vi "Untitled 4.vi"() -> ()   [LabVIEW 2021]
panel:
  out "length":i32
  out "data string":string
  out "result 2":i32
  in  "Array":string[](array[string])
  out "result":i32
  out "appended array":string[](array[string])
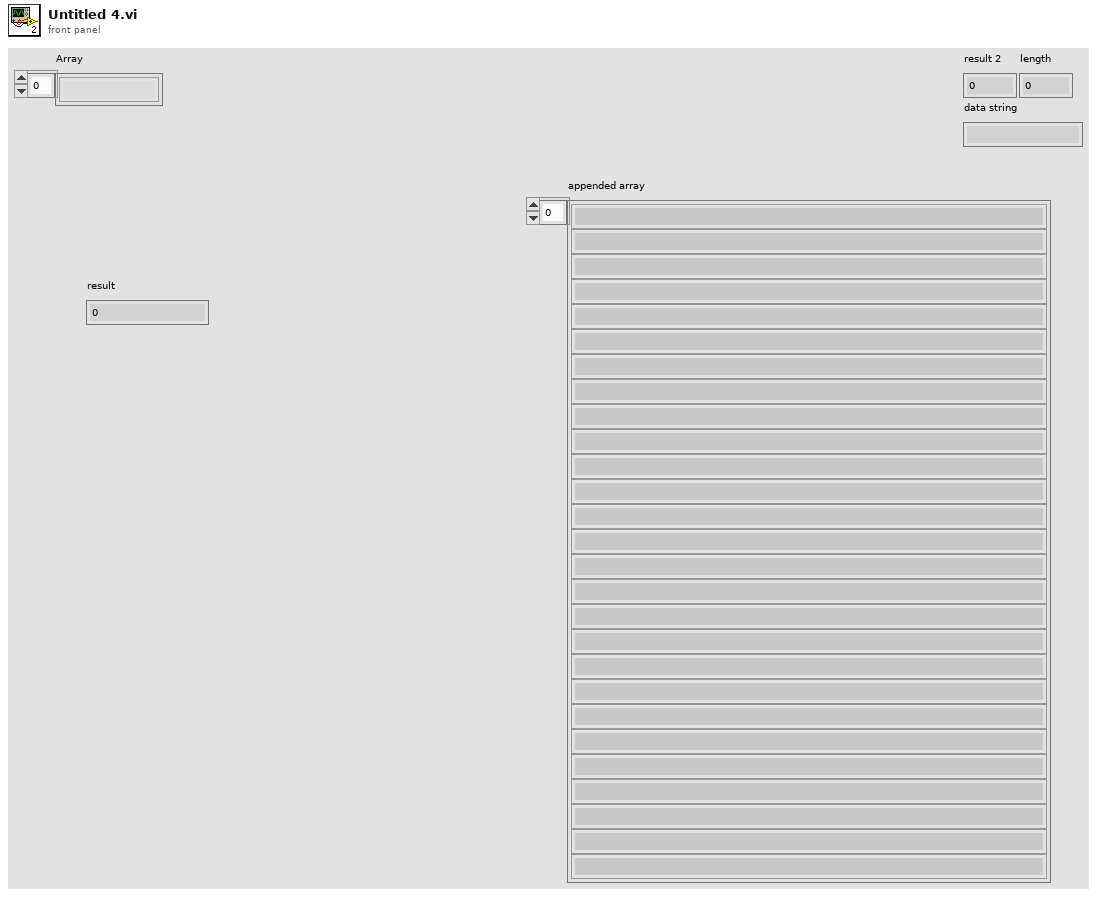
[diagram p1: front panel]
types:
  T1 = typedef "LVDateTimeRec.ctl" = cluster{"fractional second":dbl, "second":i32, "minute":i32, "hour":i32, "day of month":i32, "month":i32, "year":i32, "day of week":i32, "day of year":i32, "DST":i32}
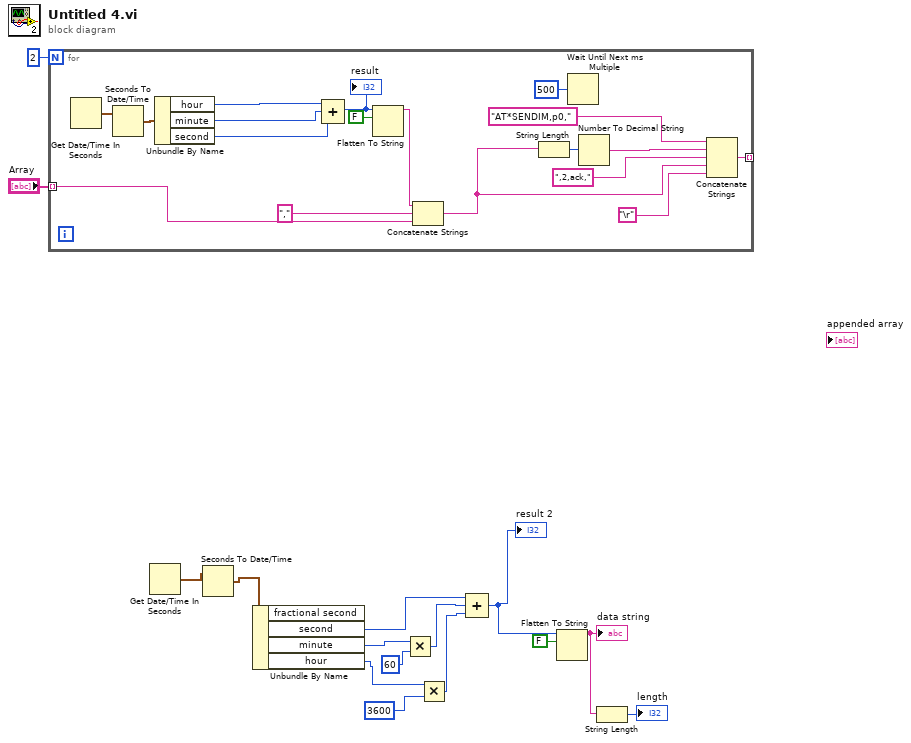
[diagram p0: block diagram]
diagram:
  n1 = for {
    N: 2 -> [_]
    tunnel: "Array" -> [w23] mode=indexing
    tunnel: [w28] -> _ mode=indexing
    n2 = Get Date/Time In Seconds() -> (seconds since 1Jan1904=w26:timestamp)
    n3 = Seconds To Date/Time(time stamp (now)=w26) -> (date time rec=w25:T1)  [unwired: 1 in]
    n4 = Unbundle By Name(w25) -> ("hour"=w22:i32, "minute"=w21:i32, "second"=w20:i32)
    n5 = Compound Arithmetic op=ADD(w22, w21, w20) -> (w19:i32)
    "result" <- w19
    n6 = Flatten To String(anything=w19, prepend array or string size? (T)=FALSE) -> (data string=w16:string)  [unwired: 2 in, 2 out]
    n7 = Concatenate Strings(w16, "," ("string"), w23) -> (w24:string)
    n8 = String Length(string=w24) -> (length=w31:i32)
    n9 = Wait Until Next ms Multiple(millisecond multiple=u32 500) -> ()  [unwired: 1 out]
    n10 = Number To Decimal String(number=w31) -> (decimal integer string=w30:string)  [unwired: 1 in]
    n11 = Concatenate Strings("AT*SENDIM,p0," ("string"), w30, ",2,ack," ("string"), w24, "\r") -> (w28:string)
  }
  n12 = Get Date/Time In Seconds() -> (seconds since 1Jan1904=w13:timestamp)
  n13 = Seconds To Date/Time(time stamp (now)=w13) -> (date time rec=w12:T1)  [unwired: 1 in]
  n14 = Unbundle By Name(w12) -> ("second"=w11:i32, "minute"=w10:i32, "hour"=w7:i32)  [unwired: 1 out]
  n15 = Multiply(x=w10, y=60) -> (x*y=w8:i32)
  n16 = Multiply(x=w7, y=3600) -> (x*y=w5:i32)
  n17 = Compound Arithmetic op=ADD(w11, w8, w5) -> (w4:i32)
  "result 2" <- w4
  n18 = Flatten To String(anything=w4, prepend array or string size? (T)=FALSE) -> (data string=w2:string)  [unwired: 2 in, 2 out]
  "data string" <- w2
  n19 = String Length(string=w2) -> (length=→"length":i32)
